vi "taskqueue ref.vi"(8 "错误输入（无错误）":errorcluster) -> (0 "错误输出":errorcluster, 3 "队列输出":refnum<queue>)   [LabVIEW 2016, in "综合生物毒性.lvlib"]
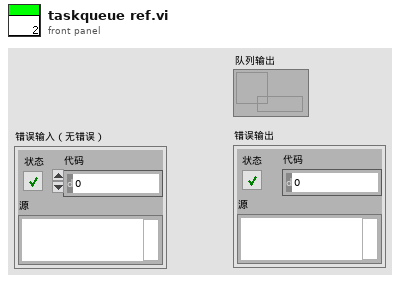
[diagram p1: front panel]
types:
  T1 = typedef "控制命令与参数.ctl" = cluster{"控制命令":enum16{"启动测量", "标样核查", "零点核查", "跨度核查", "空白测试", "平行样测试", "加标回收", "空白校准", "标样校准", "初始化（清洗）", "停止测试", "仪器重启", "校时", "模式设置", "测量间隔设置"}, "测量参数":string}
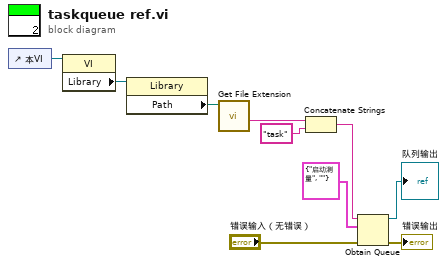
[diagram p0: block diagram]
diagram:
  n1 = control-ref of="本VI"() -> (w9:refnum<vi>)
  n2 = property class="VI"(reference=w9) -> ("Library"=w10:refnum<vi>)  [unwired: 1 in, 2 out]
  n3 = property class="Library"(reference=w10) -> ("Path"=w8:path)  [unwired: 1 in, 2 out]
  n4 = call <vilib>:"Get File Extension.vi"("file"=w8) -> ("filename without extension"=w1:string)  [unwired: 6 in, 4 out]
  n5 = Concatenate Strings(w1, "task" ("字符串")) -> (w6:string)
  n6 = Obtain Queue(name (unnamed)=w6, element data type=T1 {"控制命令"=enum."启动测量", "测量参数"=""} ("输入参数"), error in (no error)="错误输入（无错误）") -> (queue out=→"队列输出":refnum<queue>, error out=→"错误输出":errorcluster)  [unwired: 2 in, 1 out]
